vi "Overlay Major and Minor Axes.vi"(0 "Image":T2, 5 "Initial Parameters":T1(array[cluster])) -> (4 "Image Out":T2)   [LabVIEW 2011]
uses:
  <vilib>/vision/Image Controls.llb/IMAQ Image.ctl
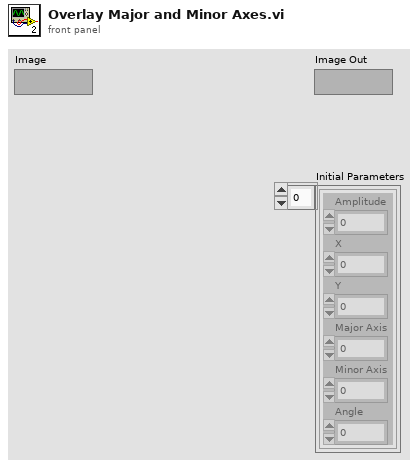
[diagram p1: front panel]
types:
  T1 = cluster{"Amplitude":dbl, "X":dbl, "Y":dbl, "Major Axis":dbl, "Minor Axis":dbl, "Angle":dbl}[]
  T2 = typedef "IMAQ Image.ctl" = refnum<image>
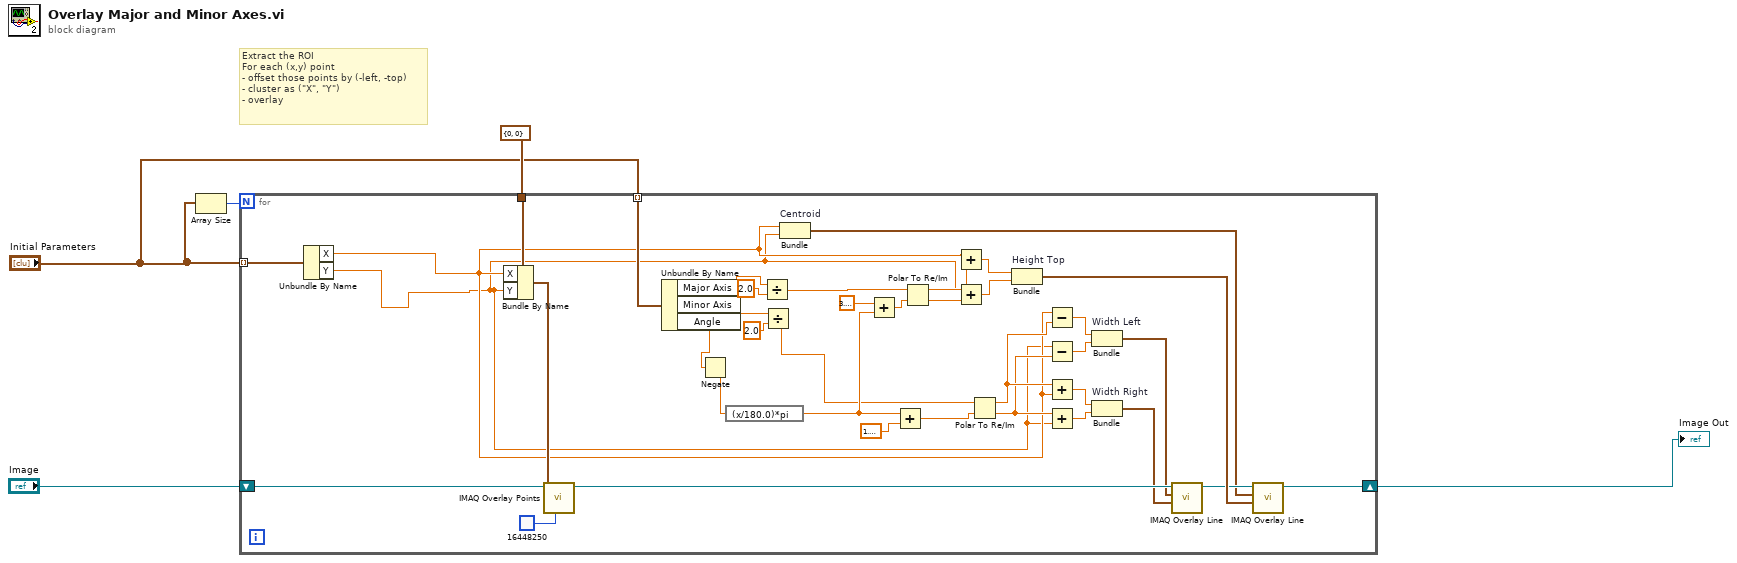
[diagram p0: block diagram]
diagram:
  # "Extract the ROI\nFor each (x,y) point\n- offset those points by (-left, -top)\n- cluster as (\"X\", \"Y\")\n- overlay"
  n1 = Array Size(array="Initial Parameters") -> (size(s)=w5:i32)
  n2 = for {
    N: w5 -> [_]
    tunnel: "Initial Parameters" -> [w39] mode=indexing
    tunnel: cluster{"X":i32, "Y":i32} {"X"=0, "Y"=0} -> [w43]
    shift-right: [w34] -> w3
    shift-left: "Image" -> [w41]
    tunnel: "Initial Parameters" -> [w25] mode=indexing
    n3 = Unbundle By Name(w39) -> ("X"=w8:dbl, "Y"=w7:dbl)
    n4 = Bundle By Name(cluster=w43, "X"=w8, "Y"=w7) -> (w42:cluster{"X":i32, "Y":i32})
    n5 = call "IMAQ Overlay Points"("Color"=u32 16448250, "Point"=w42, "Image"=w41) -> ("Image Out"=w26:T2)  [unwired: 7 in, 1 out]
    n6 = Unbundle By Name(w25) -> ("Major Axis"=w24:dbl, "Minor Axis"=w10:dbl, "Angle"=w6:dbl)
    n7 = Negate(x=w6) -> (-x=w31:dbl)
    n8 = expression code="(x/180.0)*pi" ("degrees to radians")(w31) -> (w20:dbl)
    n9 = Divide(x=w24, y=2.0) -> (x/y=w23:dbl)
    n10 = Divide(x=w10, y=2.0) -> (x/y=w11:dbl)
    n11 = Bundle "Centroid"("X"=w8, "Y"=w7) -> (w18:cluster{"X":dbl, "Y":dbl})  [unwired: 1 in]
    n12 = Add(x=3.141592653589793, y=w20) -> (x+y=w32:dbl)
    n13 = Add(x=w20, y=1.5707963267948966) -> (x+y=w21:dbl)
    n14 = Polar To Re/Im(2:w32, 3:w23) -> (0:w35:dbl, 1:w36:dbl)
    n15 = Add(x=w8, y=w36) -> (x+y=w38:dbl)
    n16 = Add(x=w7, y=w35) -> (x+y=w37:dbl)
    n17 = Polar To Re/Im(2:w21, 3:w11) -> (0:w15:dbl, 1:w16:dbl)
    n18 = Bundle "Height Top"(w38, w37) -> (w33:cluster{dbl, dbl})  [unwired: 1 in]
    n19 = Subtract(x=w8, y=w16) -> (x-y=w14:dbl)
    n20 = Subtract(x=w7, y=w15) -> (x-y=w13:dbl)
    n21 = Add(x=w16, y=w8) -> (x+y=w29:dbl)
    n22 = Add(x=w15, y=w7) -> (x+y=w28:dbl)
    n23 = Bundle "Width Left"(w14, w13) -> (w12:cluster{dbl, dbl})  [unwired: 1 in]
    n24 = Bundle "Width Right"(w29, w28) -> (w17:cluster{dbl, dbl})  [unwired: 1 in]
    n25 = call "IMAQ Overlay Line"("End Point"=w17, "Start Point"=w12, "Image"=w26) -> ("Image Out"=w27:T2)  [unwired: 7 in, 1 out]
    n26 = call "IMAQ Overlay Line"("End Point"=w33, "Start Point"=w18, "Image"=w27) -> ("Image Out"=w34:T2)  [unwired: 7 in, 1 out]
  }
  "Image Out" <- w3
